vi "Dynamixel Motor Send Advanced Commands.vi"() -> ()   [LabVIEW 2016]
doc: "This example allows you to use all of the available command types for the Dynamixel motor. Refer to the motor's documentation for more information."
uses:
  <instrlib>/Dynamixel Motor/Public/Motor Operation/Low Level/Baud Setting.ctl
  <instrlib>/Dynamixel Motor/Dynamixel Motor.lvlib
panel:
  in  "Force Baud Rate (True)":bool=TRUE
  out "Last command sent":string
  in  "Select Action":u16(ring) items=["Ping", "Read", "Write", "Registered Write", "Action", "Reset", "Sync Write"]
  in  "Baud rate (57600 bps)":T1=34 items=["1,000,000 bps"=1, "500,000 bps"=3, "400,000 bps"=4, "250,000 bps"=7, "200,000 bps"=9, "115200 bps"=16, "57600 bps"=34, "19200 bps"=103, "9600 bps"=207]
  in  "VISA resource name":refnum<visa-resource-name>
  in  "stop":bool
  out "Responses":string
  in  "Send Command":bool
  in  "Parameters (Hex)":string
  in  "Address":u8
  in  "Motor ID":u8
  in  "Clear":bool
  # "(c) 2011-2012  National Instruments.  ALL RIGHTS RESERVED."
  # "This example allows you to use all of the available command types for the \nDynamixel motor.  Refer to the motor's documentation for more information."
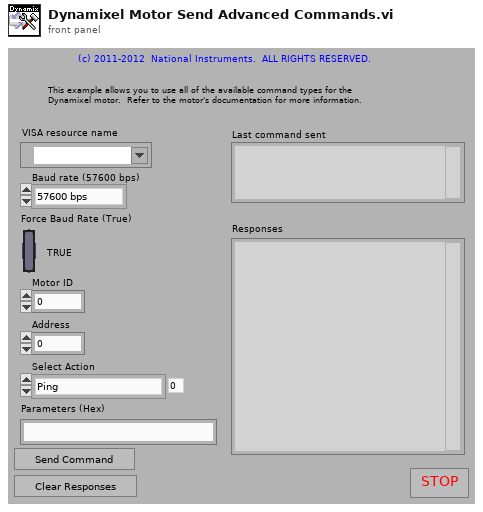
[diagram p1: front panel]
types:
  T1 = typedef "Dynamixel Motor.lvlib/Baud Setting.ctl" = u8
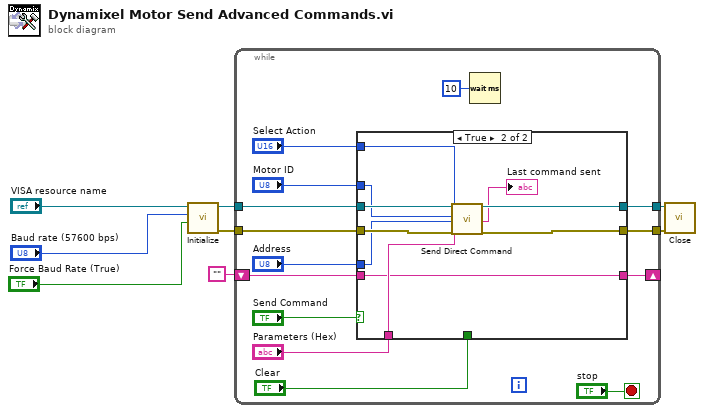
[diagram p0: block diagram]
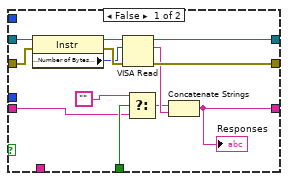
[diagram p2: hidden frame]
diagram:
  n1 = call <instrlib>:"Initialize.vi"("Force Baud Rate (True)"="Force Baud Rate (True)", "Baud rate (57600 bps)"="Baud rate (57600 bps)", "VISA resource name"="VISA resource name") -> ("error out"=w7:errorcluster, "VISA resource name out"=w3:refnum<visa-resource-name>)  [unwired: 7 in]
  n2 = while {
    tunnel: w3 -> [w22]
    tunnel: [w21] -> w8
    tunnel: w7 -> [w20]
    tunnel: [w19] -> w6
    shift-right: [w10] -> _
    shift-left: "" -> [w9]
    stop <- "stop" stop-if-true
    n3 = case shown="True" "Send Command" {
      tunnel: w22 -> [w35 w45]
      tunnel: [w30 w44] -> w21
      tunnel: w20 -> [w34 w43]
      tunnel: [w29 w42] -> w19
      tunnel: "Parameters (Hex)" -> [_ w41]
      tunnel: "Address" -> [_ w40]
      tunnel: "Motor ID" -> [_ w39]
      tunnel: "Clear" -> [w27 _]
      tunnel: "Select Action" -> [_ w38]
      tunnel: [w24 w36] -> w10
      tunnel: w9 -> [w23 w36]
      frame False {
        n4 = property class="Instr"(reference=w35, error in=w34) -> (reference out=w31:refnum<visa-resource-name>, error out=w33:errorcluster, "Serial Settings:Number of Bytes at Serial Port"=w32:u32)
        n5 = VISA Read(VISA resource name=w31, byte count=w32, error in (no error)=w33) -> (VISA resource name out=w30:refnum<visa-resource-name>, read buffer=w28:string, error out=w29:errorcluster)  [unwired: 1 out]
        n6 = Select(t="", s=w27, f=w23) -> (s? t:f=w26:string)
        n7 = Concatenate Strings(w26, w28) -> (w24:string)
        "Responses" <- w24
      }
      frame True {
        n8 = call <instrlib>:"Send Direct Command.vi"("VISA resource name"=w45, "Select Action"=w38, "Motor ID (0)"=w39, "Address"=w40, "Parameters"=w41, "Error in (no error)"=w43) -> ("VISA resource name out"=w44:refnum<visa-resource-name>, "Command to Serial"=→"Last command sent":string, "Error out"=w42:errorcluster)  [unwired: 11 in]
      }
    }
    n9 = Wait (ms)(milliseconds to wait=u32 10) -> ()  [unwired: 1 out]
  }
  n10 = call <instrlib>:"Close.vi"("error in (no error)"=w6, "VISA resource name"=w8) -> ()  [unwired: 9 in, 1 out]
